vi "SQL_Table_Warning_Record_Insert.vi"(10 "时间":string, 11 "报警信息":T1) -> (3 "error out":errorcluster)   [LabVIEW 2014]
uses:
  Terminal_Global_TestID.vi
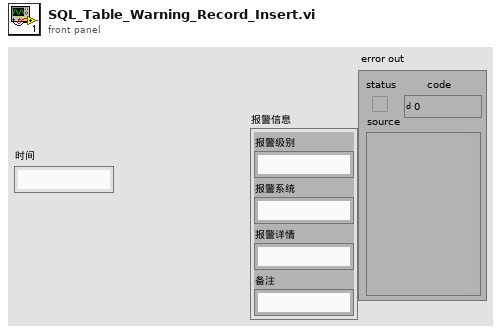
[diagram p1: front panel]
types:
  T1 = cluster{"报警级别":string, "报警系统":string, "报警详情":string, "备注":string}
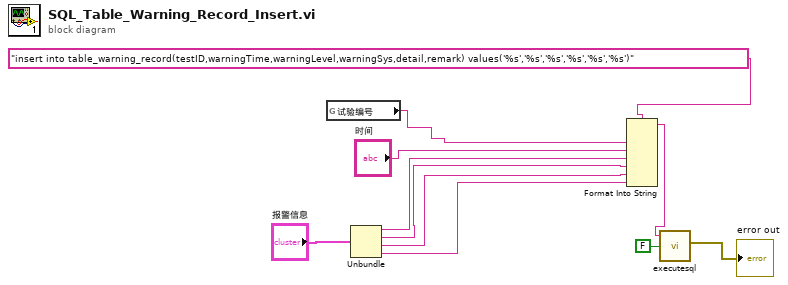
[diagram p0: block diagram]
diagram:
  n1 = global read "Terminal_Global_TestID.vi" "试验编号"() -> (w1:string)
  n2 = Unbundle("报警信息") -> ("报警级别"=w7:string, "报警系统"=w6:string, "报警详情"=w5:string, "备注"=w4:string)
  n3 = Format Into String(format string="insert into table_warning_record(testID,warningTime,warningLevel,warningSys,detail,remark) values('%s','%s','%s','%s','%s','%s')" ("Command Text"), w1, "时间", w7, w6, w5, w4) -> (resulting string=w3:string)  [unwired: 2 in, 1 out]
  n4 = call "executesql.vi"("Return Data (T)"=FALSE, "Command Text"=w3) -> ("error out"=→"error out":errorcluster)  [unwired: 5 in, 1 out]
